vi "Extract String Values (SubVI).vi"(10 "Communication":enum16{"TCP", "GPIB"}(ring), 11 "read buffer":string) -> (3 "array type (2D Dbl)":dbl[](array[numeric]))   [LabVIEW 2021]
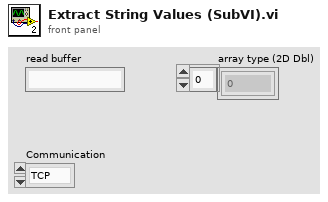
[diagram p1: front panel]
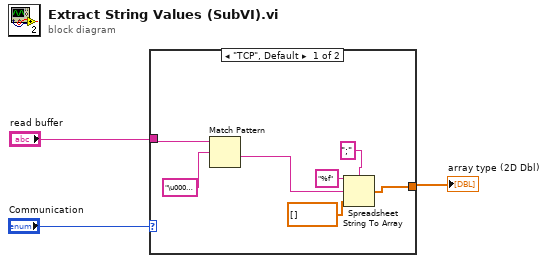
[diagram p0: block diagram]
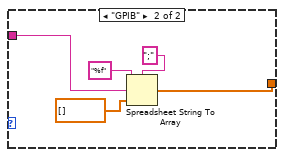
[diagram p2: hidden frame]
diagram:
  n1 = case shown="\"TCP\", Default" "Communication" {
    tunnel: "read buffer" -> [w6 w13]
    tunnel: [w8 w12] -> w2
    frame "TCP", Default {
      n2 = Match Pattern(string=w6, regular expression="\u0000\u0000\u0000\u0000I\u0000\u0000\u0000 ") -> (after substring=w5:string)  [unwired: 1 in, 3 out]
      n3 = Spreadsheet String To Array(delimiter (Tab)=";", format string="%f", spreadsheet string=w5, array type (2D Dbl)=dbl[] []) -> (array=w8:dbl[])
    }
    frame "GPIB" {
      n4 = Spreadsheet String To Array(delimiter (Tab)=";", format string="%f", spreadsheet string=w13, array type (2D Dbl)=dbl[] []) -> (array=w12:dbl[])
    }
  }
  "array type (2D Dbl)" <- w2
